vi "BroadCast Server.vi"(0 "Information Package":string, 5 "TCP Server":refnum<k5>) -> ()   [LabVIEW 2017, in "CL_G3_BuilderApplicationLayer.lvlib"]
uses:
  CL_G3_BuilderApplicationLayer.lvlib
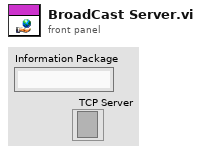
[diagram p1: front panel]
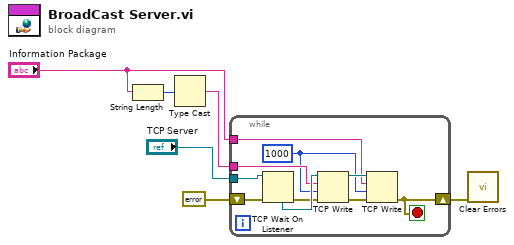
[diagram p0: block diagram]
diagram:
  n1 = String Length(string="Information Package") -> (length=w5:i32)
  n2 = Type Cast(x=w5) -> (*(type *) &x=w6:string)  [unwired: 1 out]
  n3 = while {
    tunnel: w6 -> [w11]
    tunnel: "Information Package" -> [w10]
    shift-right: [w7] -> w4
    shift-left: errorcluster {"status"=FALSE, "code"=0, "source"=""} ("error out") -> [w15]
    tunnel: "TCP Server" -> [w16]
    stop <- w7 stop-if-true
    w8 = 1000 ("timeout ms (25000)")
    n4 = TCP Wait On Listener(8:w15, 11:w16) -> (0:w9:errorcluster, 4:w12:refnum<k5>)  [unwired: 2 in, 3 out]
    n5 = TCP Write(connection ID=w12, data in=w11, error in (no error)=w9, 9:w8) -> (connection ID out=w14:refnum<k5>, error out=w13:errorcluster)  [unwired: 1 out]
    n6 = TCP Write(connection ID=w14, data in=w10, error in (no error)=w13, 9:w8) -> (error out=w7:errorcluster)  [unwired: 2 out]
  }
  n7 = call <vilib>:"Clear Errors.vi"("error in (no error)"=w4) -> ()  [unwired: 5 in, 2 out]
